vi "CODCr数据插入DATA (子VI).vi"(11 "Enum输入":refnum<vi>) -> (3 "data":T1)   [LabVIEW 2016, in "CODCr库.lvlib"]
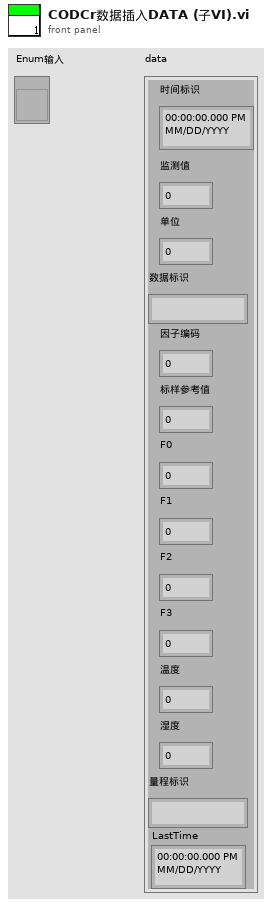
[diagram p1: front panel]
types:
  T1 = cluster{"时间标识":timestamp, "监测值":sgl, "单位":u16, "数据标识":string, "因子编码":u32, "标样参考值":sgl, "F0":sgl, "F1":sgl, "F2":sgl, "F3":sgl, "温度":sgl, "湿度":sgl, "量程标识":string, "LastTime":timestamp}
  T2 = cluster{"因子编码":u32, "单位":u16, "标样参考值":sgl, "水样数据时间":timestamp, "水样实测值":sgl, "水样数据标识":string, "标样数据时间":timestamp, "标样实测值":sgl, "标样数据标识":string, "空白数据时间":timestamp, "空白实测值":sgl, "空白数据标识":string, "零点核查数据时间":timestamp, "零点核查实测值":sgl, "零点核查数据标识":string, "跨度核查数据时间":timestamp, "跨度核查实测值":sgl, "跨度核查数据标识":string, "加标回收数据时间":timestamp, "加标回收实测值":sgl, "加标回收数据标识":string, "平行样数据时间":timestamp, "平行样实测值":sgl, "平行样数据标识":string}
  T3 = cluster{"系统时间":timestamp, "工作状态":u16, "测量模式":u16, "告警代码":u16, "故障代码":u16, "日志代码":u16, "软件版本":u16, "F0":sgl, "F1":sgl, "F2":sgl, "F3":sgl, "T":sgl, "H":sgl, "id":u16, "flowid":u16, "量程":u16}
  T4 = cluster{"跨度值":dbl, "零点标准液浓度":dbl, "跨度标准液浓度":dbl, "标准液标准浓度":dbl}
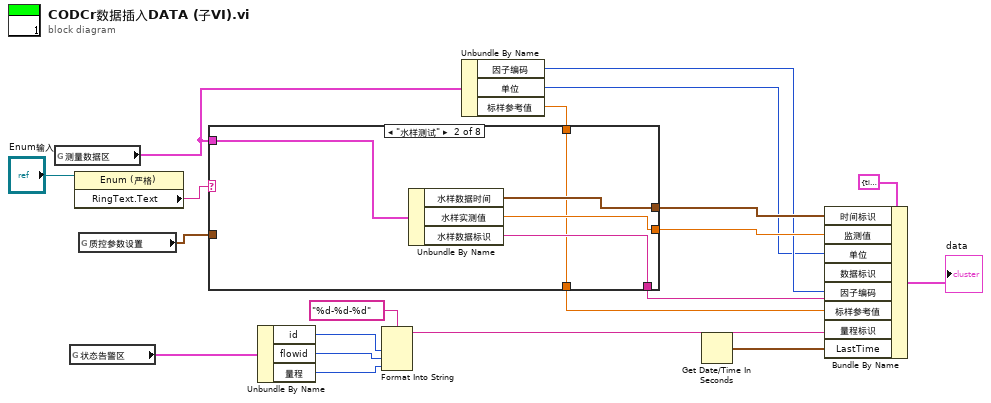
[diagram p0: block diagram]
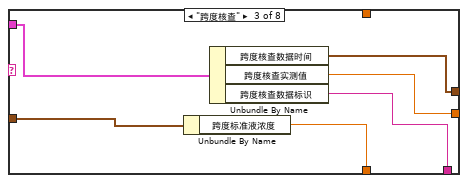
[diagram p3: hidden frame]
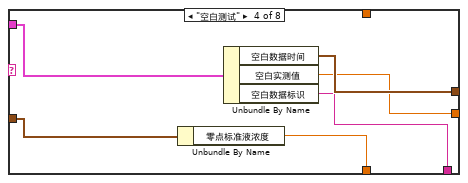
[diagram p4: hidden frame]
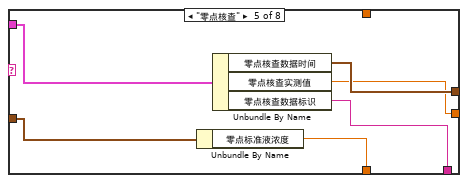
[diagram p5: hidden frame]
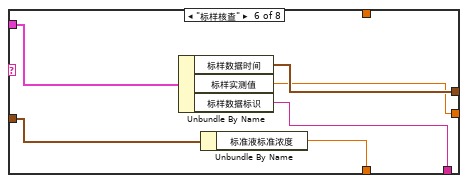
[diagram p6: hidden frame]
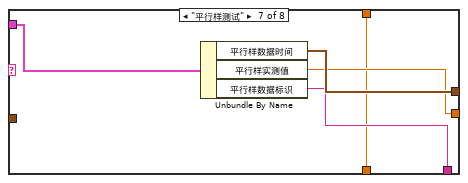
[diagram p7: hidden frame]
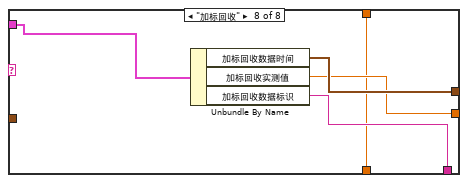
[diagram p8: hidden frame]
diagram:
  n1 = global read "CODcr全局变量.vi" "测量数据区"() -> (w7:T2)
  n2 = global read "CODcr全局变量.vi" "状态告警区"() -> (w8:T3)
  n3 = property on="属性节点" class="Enum (严格)"(reference="Enum输入") -> ("RingText.Text"=w10:string)  [unwired: 1 in, 2 out]
  n4 = global read "CODcr全局变量.vi" "质控参数设置"() -> (w1:T4)
  n5 = Unbundle By Name(w8) -> ("id"=w14:u16, "flowid"=w15:u16, "量程"=w16:u16)
  n6 = Format Into String(format string="%d-%d-%d" ("格式字符串"), w14, w15, w16) -> (resulting string=w17:string)  [unwired: 2 in, 1 out]
  n7 = Unbundle By Name(w7) -> ("因子编码"=w12:u32, "单位"=w11:u16, "标样参考值"=w3:sgl)
  n8 = case shown="\"水样测试\"" w10 {
    tunnel: w7 -> [_ w26 w32 w38 w44 w47 w52 w57]
    tunnel: [_ w25 w31 w37 w43 w50 w55 w60] -> w18
    tunnel: [_ w24 w30 w36 w42 w49 w54 w59] -> w19
    tunnel: [_ w23 w29 w35 w41 w48 w53 w58] -> w20
    tunnel: w3 -> [w21 w22 _ _ _ _ w51 w56]
    tunnel: [w21 w22 w27 w34 w40 w46 w51 w56] -> w2
    tunnel: w1 -> [_ _ w28 w33 w39 w45 _ _]
    frame "假", Default {
    }
    frame "水样测试" {
      n9 = Unbundle By Name(w26) -> ("水样数据时间"=w25:timestamp, "水样实测值"=w24:sgl, "水样数据标识"=w23:string)
    }
    frame "跨度核查" {
      n10 = Unbundle By Name(w28) -> ("跨度标准液浓度"=w27:dbl)
      n11 = Unbundle By Name(w32) -> ("跨度核查数据时间"=w31:timestamp, "跨度核查实测值"=w30:sgl, "跨度核查数据标识"=w29:string)
    }
    frame "空白测试" {
      n12 = Unbundle By Name(w33) -> ("零点标准液浓度"=w34:dbl)
      n13 = Unbundle By Name(w38) -> ("空白数据时间"=w37:timestamp, "空白实测值"=w36:sgl, "空白数据标识"=w35:string)
    }
    frame "零点核查" {
      n14 = Unbundle By Name(w39) -> ("零点标准液浓度"=w40:dbl)
      n15 = Unbundle By Name(w44) -> ("零点核查数据时间"=w43:timestamp, "零点核查实测值"=w42:sgl, "零点核查数据标识"=w41:string)
    }
    frame "标样核查" {
      n16 = Unbundle By Name(w47) -> ("标样数据时间"=w50:timestamp, "标样实测值"=w49:sgl, "标样数据标识"=w48:string)
      n17 = Unbundle By Name(w45) -> ("标准液标准浓度"=w46:dbl)
    }
    frame "平行样测试" {
      n18 = Unbundle By Name(w52) -> ("平行样数据时间"=w55:timestamp, "平行样实测值"=w54:sgl, "平行样数据标识"=w53:string)
    }
    frame "加标回收" {
      n19 = Unbundle By Name(w57) -> ("加标回收数据时间"=w60:timestamp, "加标回收实测值"=w59:sgl, "加标回收数据标识"=w58:string)
    }
  }
  n20 = Get Date/Time In Seconds() -> (seconds since 1Jan1904=w4:timestamp)
  n21 = Bundle By Name(cluster=T1 {"时间标识"=timestamp(0 s since 1904-01-01), "监测值"=0.0, "单位"=0, "数据标识"="", "因子编码"=0, "标样参考值"=0.0, "F0"=0.0, "F1"=0.0, "F2"=0.0, "F3"=0.0, "温度"=0.0, "湿度"=0.0, "量程标识"="", "LastTime"=timestamp(0 s since 1904-01-01)} ("data"), "时间标识"=w18, "监测值"=w19, "单位"=w11, "数据标识"=w20, "因子编码"=w12, "标样参考值"=w2, "量程标识"=w17, "LastTime"=w4) -> (→"data":T1)
